vi "alignment_server_zmq.vi"() -> ()   [LabVIEW 2012]
uses:
  <vilib>/Platform/TimedLoop/XDataNode/wakeup.ctl
  <vilib>/Platform/TimedLoop/XDataNode/XDNodeRunTimeDep.lvlib
  <vilib>/Platform/TimedLoop/XDataNode/nitl_modes.ctl
  <vilib>/Platform/TimedLoop/XDataNode/timing_clust.ctl
  <vilib>/platform/TimedLoop/XDataNode/XDataNode.xnode
  Analog_Input/Analog_Input.lvclass
  PicoMotor.lvclass
  picomotor_control_array.ctl
  NewFocus8742/Command VIs/picomotor_control.ctl
  <vilib>/addons/zeromq/socket_type.ctl
panel:
  in  "enable":bool[](array[boolean])=[TRUE, TRUE, TRUE, TRUE]
  out "stopped?":bool[](array[boolean])
  out "Actual Positions":i32[](array[numeric])
  in  "Set Positions":i32[](array[numeric])=[0, 0, 0, 0] step=10
  in  "samples per channel":i32=100
  out "RECV'd message":string
  in  "Picomotor controls":T1=[{"enable"=TRUE, "description"="x1", "Set Position "=0, "Actual Position"=0, "stopped?"=TRUE, "zero"=FALSE, "Motor Type"=3, "Steps/s"=1750, "Steps/s^2"=100000}, {"enable"=TRUE, "description"="x2", "Set Position "=0, "Actual Position"=0, "stopped?"=TRUE, "zero"=FALSE, "Motor Type"=3, "Steps/s"=1750, "Steps/s^2"=100000}, {"enable"=TRUE, "description"="x3", "Set Position "=0, "Actual Position"=0, "stopped?"=TRUE, "zero"=FALSE, "Motor Type"=3, "Steps/s"=1750, "Steps/s^2"=100000}, {"enable"=TRUE, "description"="x4", "Set Position "=0, "Actual Position"=0, "stopped?"=TRUE, "zero"=FALSE, "Motor Type"=3, "Steps/s"=1750, "Steps/s^2"=100000}] {"Motor Type" items=["NoMotor", "Undefined", "Tiny", "Standard"]; "Set Position" step=100}
  in  "shutdown":bool caption="quit"
  in  "halt":bool caption="quit"
  out "voltage":dbl[](array[numeric])=[1.3462267936011734]
  out "coupling chart":dbl(graph)
  in  "descriptions":string[](array[string])
  out "DeviceKey Out":string="8742 10116"
  in  "sample rate (Hz)":dbl=1000.0
  in  "physical channels":tag="PXI1Slot7/ai0"
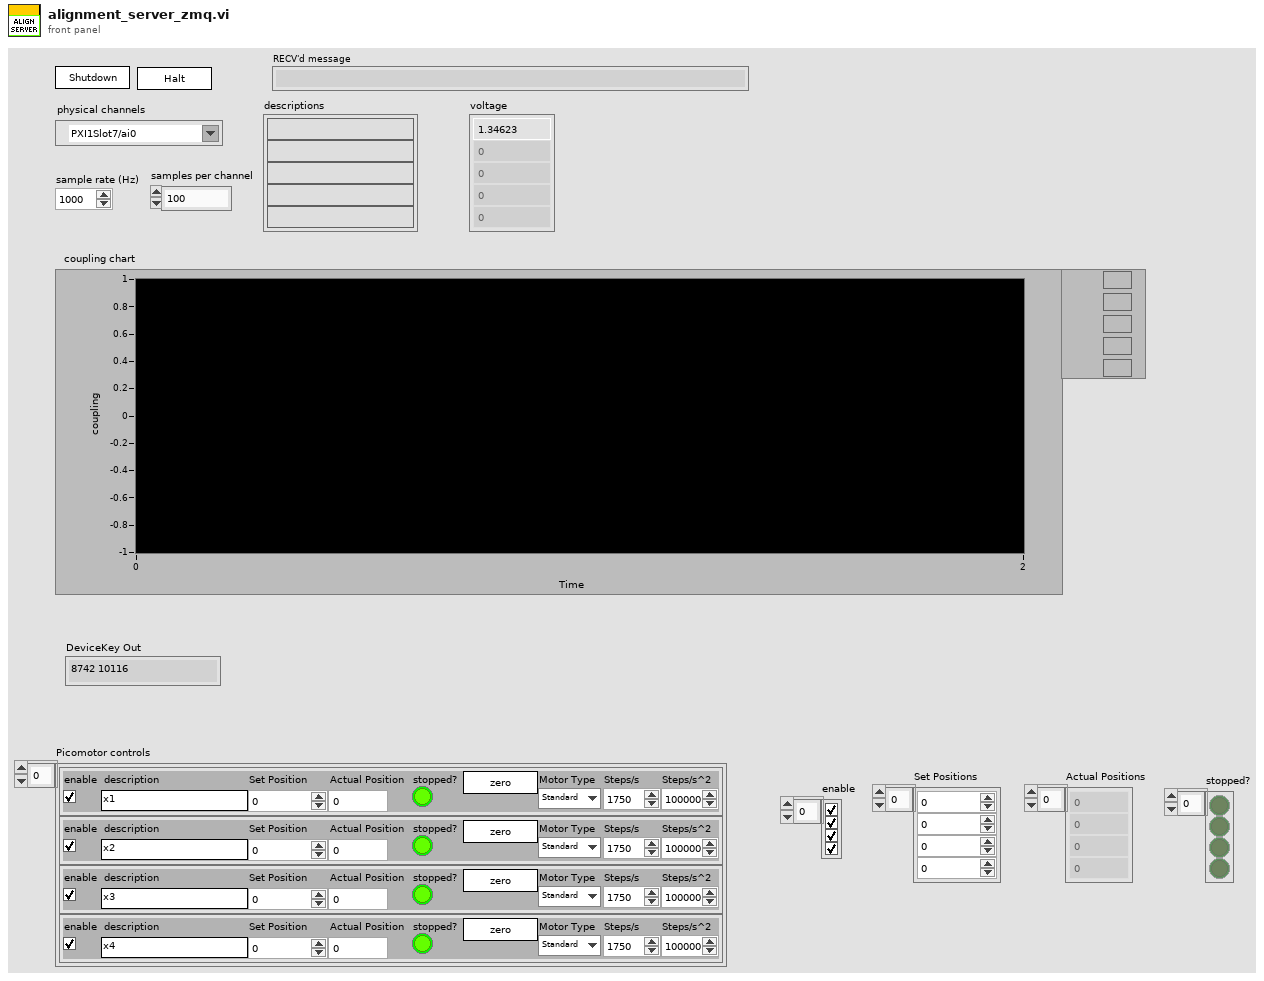
[diagram p1: front panel]
types:
  T1 = typedef "PicoMotor.lvclass/picomotor_control_array.ctl" = T2[]
  T2 = typedef "PicoMotor.lvclass/picomotor_control.ctl" = cluster{"enable":bool, "description":string, "Set Position ":i32, "Actual Position":i32, "stopped?":bool, "zero":bool, "Motor Type":i32, "Steps/s":i32, "Steps/s^2":i32}
  T3 = typedef "zeromq.lvlib/socket_type.ctl" = enum8{"ZMQ_PAIR", "ZMQ_PUB", "ZMQ_SUB", "ZMQ_REQ", "ZMQ_REP", "ZMQ_DEALER", "ZMQ_ROUTER", "ZMQ_PULL", "ZMQ_PUSH", "ZMQ_XPUB", "ZMQ_XSUB"}
  T4 = typedef "XDNodeRunTimeDep.lvlib/timing_clust.ctl" = cluster{"Expected End [f-1]":u64, "Actual End [f-1]":u64, "Finished Late? [f-1]":bool, "Expected End [i-1]":u64, "Actual End [i-1]":u64, "Finished Late? [i-1]":bool, "Expected Start [i]":u64, "Actual Start [i]":u64, "Expected Start [f]":u64, "Actual Start [f]":u64, "Source Name":string, "Structure Name":string, "Period":i64, "Deadline":i64, "Offset":i64, "Start":i64, "Priority":i32, "Timeout":i32, "Mode":T5, "Wakeup Reason":T6, "Error":errorcluster, "Source Type":string, "Secondary Source Type":string, "Global End Time":u64, "Global Start Time":u64, "Frame Duration":u64, "Iteration Duration":u64, "Assigned CPU":i32, "I/O Scan Engine Mode":u32}
  T5 = typedef "XDNodeRunTimeDep.lvlib/nitl_modes.ctl" = enum32{"No Change", "Process missed periods, maintain original phase", "Discard missed periods, maintain original phase", "Process missed periods, ignore original phase", "Discard missed periods, ignore original phase"}
  T6 = typedef "XDNodeRunTimeDep.lvlib/wakeup.ctl" = enum32{"Normal", "Aborted", "Asynchronous wakeup", "Timing source error", "Timed loop error", "Timeout"}
  T7 = typedef "pointer.ctl" = u64
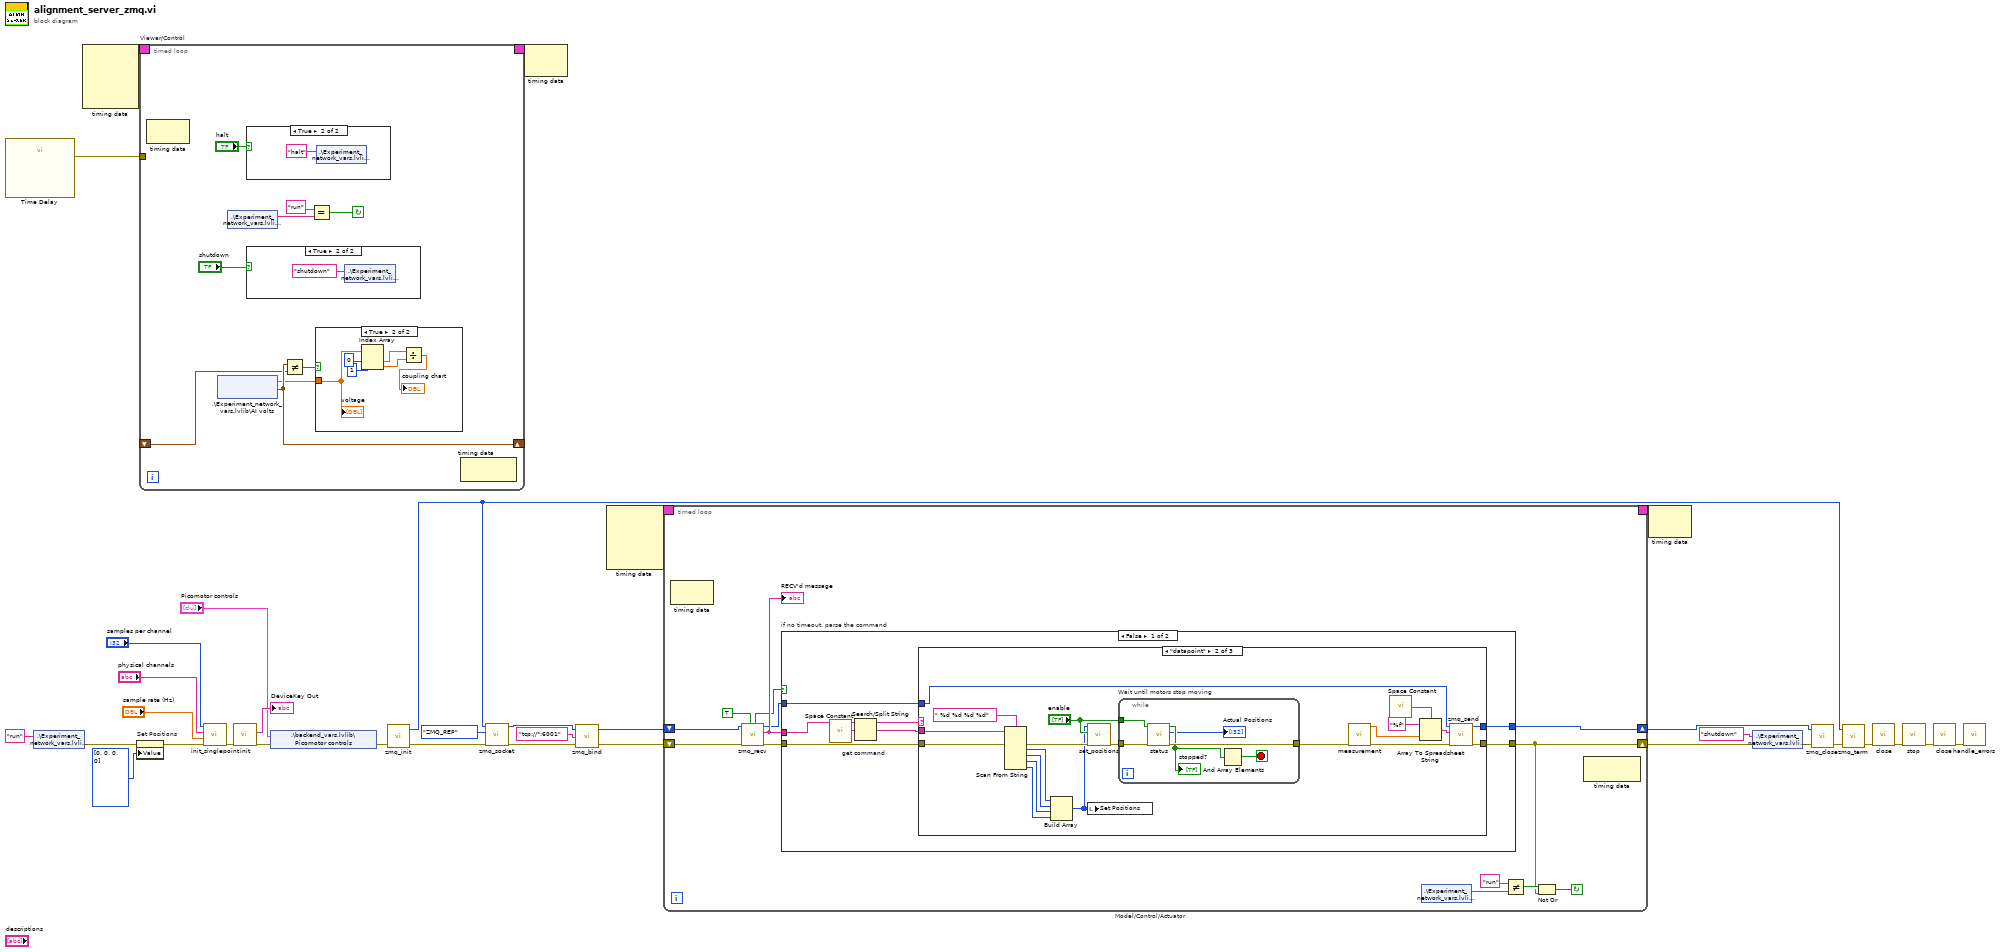
[diagram p0: block diagram]
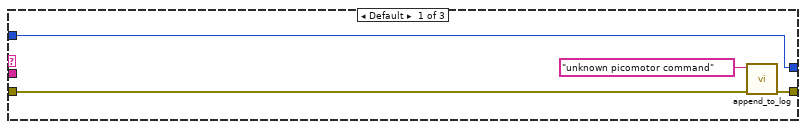
[diagram p2: hidden frame]
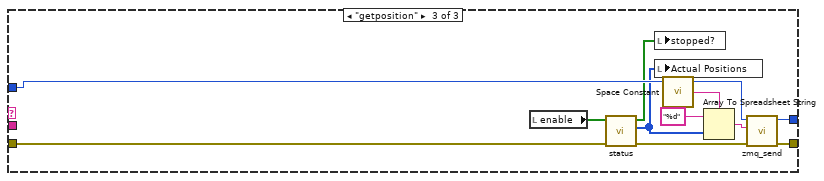
[diagram p3: hidden frame]
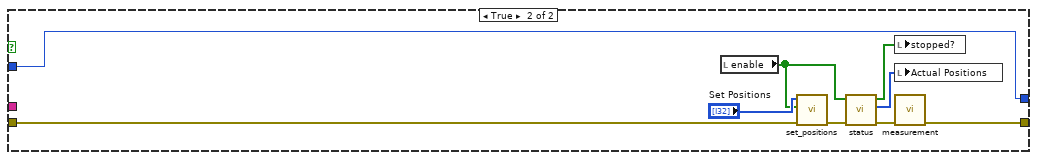
[diagram p4: hidden frame]
diagram:
  n1 = call "Time Delay"() -> ("error out"=w8:errorcluster)  [unwired: 11 in]
  n2 = shared-variable ".\\Experiment_network_vars.lvlib\\state"("run" ("state")) -> (error out=w3:errorcluster)  [unwired: 1 in]
  n3 = node-c288() -> (w34:T4)  [unwired: 4 in]
  n4 = property on="Set Positions" class="Arr (strict)"(error in=w3, "Value"=i32[] [0, 0, 0, 0] ("Set Positions")) -> (error out=w2:errorcluster)  [unwired: 1 in, 1 out]
  n5 = timed-loop "Viewer/Control" {
    timing: w34 -> [_]
    timing-out: [_] -> w33
    tunnel: w8 -> [_]
    shift-right: [w38] -> _
    shift-left: _ -> [w37]
    stop <- w39 continue-if-true
    n6 = node-c288() -> ()  [unwired: 1 in, 1 out]
    n7 = shared-variable ".\\Experiment_network_vars.lvlib\\AI volts"() -> (w35:dbl[], w38:timestamp)  [unwired: 1 in, 1 out]
    n8 = shared-variable ".\\Experiment_network_vars.lvlib\\state"() -> (w41:string)  [unwired: 1 in, 1 out]
    n9 = case shown="True" "halt" {
      frame False {
      }
      frame True {
        n10 = shared-variable ".\\Experiment_network_vars.lvlib\\state"("halt" ("state")) -> ()  [unwired: 1 in, 1 out]
      }
    }
    n11 = case shown="True" "shutdown" {
      frame False {
      }
      frame True {
        n12 = shared-variable ".\\Experiment_network_vars.lvlib\\state"("shutdown" ("state")) -> ()  [unwired: 1 in, 1 out]
      }
    }
    n13 = Not Equal?(x=w38, y=w37) -> (x != y?=w36:bool)
    n14 = Equal?(x="run", y=w41) -> (x = y?=w39:bool)
    n15 = case shown="True" w36 {
      tunnel: w35 -> [_ w48]
      frame False {
      }
      frame True {
        n16 = Index Array(array=w48, index #1=0 ("index"), index #2=1 ("index")) -> (element #1=w46:dbl, element #2=w45:dbl)
        n17 = Divide(x=w46, y=w45) -> (x/y=→"coupling chart":dbl)
        "voltage" <- w48
      }
    }
    n18 = node-c288() -> ()  [unwired: 1 in, 1 out]
  }
  n19 = call "init_singlepoint.vi"("error in"=w2, "sample rate (Hz)"="sample rate (Hz)", "physical channels"="physical channels", "samples per channel"="samples per channel") -> ("error out"=w5:errorcluster)  [unwired: 7 in]
  n20 = call "init.vi"("error in (no error)"=w5) -> ("error out"=w18:errorcluster, "DeviceKey"=→"DeviceKey Out":string)  [unwired: 9 in]
  n21 = shared-variable ".\\backend_vars.lvlib\\Picomotor controls"("Picomotor controls", error in=w18) -> (error out=w16:errorcluster)
  n22 = call <vilib>:"zmq_init.vi"("error in"=w16) -> ("error out"=w25:errorcluster, "context"=w23:T7)  [unwired: 3 in]
  n23 = call <vilib>:"zmq_socket.vi"("error in"=w25, "socket type"=socket_type."ZMQ_REP", "ctx in"=w23) -> ("error out"=w12:errorcluster, "socket"=w10:T7)  [unwired: 3 in]
  n24 = node-c288(w33) -> ()  [unwired: 1 out]
  n25 = call <vilib>:"zmq_bind.vi"("error in"=w12, "endpoint"="tcp://*:6001", "socket in"=w10) -> ("error out"=w11:errorcluster, "socket out"=w9:T7)  [unwired: 1 in]
  n26 = node-c288() -> (w32:T4)  [unwired: 4 in]
  n27 = timed-loop "Model/Control/Actuator" {
    timing: w32 -> [_]
    timing-out: [_] -> w31
    shift-right: [w62] -> w20
    shift-left: w9 -> [w61]
    shift-right: [w54] -> w14
    shift-left: w11 -> [w66]
    stop <- w57 continue-if-true
    n28 = node-c288() -> ()  [unwired: 1 in, 1 out]
    n29 = call <vilib>:"zmq_recv.vi"("no block? (F)"=TRUE, "error in"=w66, "socket in"=w61) -> ("error out"=w55:errorcluster, "data"=w64:string, "socket out"=w63:T7, "timeout?"=w56:bool)  [unwired: 2 in, 1 out]
    "RECV'd message" <- w64
    n30 = case "if no timeout, parse the command" shown="False" w56 {
      tunnel: [w71 w124] -> w54
      tunnel: w64 -> [w73 _]
      tunnel: w63 -> [w69 w123]
      tunnel: [w68 w123] -> w62
      tunnel: w55 -> [w67 w119]
      frame False {
        n31 = call <vilib>:"Space Constant.vi"() -> ("String"=w74:string)
        n32 = Search/Split String "get command"(string=w73, search string/char (-)=w74) -> (substring before match=w72:string, match + rest of string=w70:string)  [unwired: 1 in, 1 out]
        n33 = case shown="\"datapoint\"" w72 {
          tunnel: w67 -> [w77 w96 w115]
          tunnel: [w76 w88 w109] -> w71
          tunnel: w70 -> [_ w97 _]
          tunnel: w69 -> [w75 w90 w111]
          tunnel: [w75 w89 w108] -> w68
          frame Default {
            n34 = call "append_to_log.vi"("error in"=w77, "string"="unknown picomotor command") -> ("error out"=w76:errorcluster)  [unwired: 8 in, 1 out]
          }
          frame "datapoint" {
            n35 = Scan From String(format string=" %d %d %d %d", input string=w97, error in=w96) -> (error out=w81:errorcluster, output 1=w95:i32, output 2=w94:i32, output 3=w93:i32, output 4=w92:i32)  [unwired: 5 in, 2 out]
            n36 = Build Array(w95, w94, w93, w92) -> (w79:i32[])
            n37 = call "set_positions.vi"("error IO"=w81, "enables"="enable", "set positions"=w79) -> ("error out"=w82:errorcluster)  [unwired: 8 in]
            n38 = local write "Set Positions"(w79) -> ()
            n39 = while "Wait until motors stop moving" {
              tunnel: w82 -> [w104]
              tunnel: [w102] -> w91
              tunnel: "enable" -> [w101]
              stop <- w103 stop-if-true
              n40 = call "status.vi"("error IO"=w104, "enable"=w101) -> ("error out"=w102:errorcluster, "Actual Positions"=→"Actual Positions":i32[], "stopped?"=w100:bool[])  [unwired: 7 in]
              "stopped?" <- w100
              n41 = And Array Elements(Boolean array=w100) -> (logical AND=w103:bool)
            }
            n42 = call "measurement.vi"("error in"=w91) -> ("AI Volts"=w87:dbl[], "error out"=w83:errorcluster)  [unwired: 13 in]
            n43 = call <vilib>:"Space Constant.vi"() -> ("String"=w85:string)
            n44 = Array To Spreadsheet String(delimiter (Tab)=w85, array=w87, 3:"%f" ("format string")) -> (spreadsheet string=w84:string)
            n45 = call <vilib>:"zmq_send.vi"("error in"=w83, "data"=w84, "socket in"=w90) -> ("error out"=w88:errorcluster, "socket out"=w89:T7)  [unwired: 4 in]
          }
          frame "getposition" {
            n46 = local read "enable"() -> (w107:bool[])
            n47 = call "status.vi"("error IO"=w115, "enable"=w107) -> ("error out"=w110:errorcluster, "Actual Positions"=w105:i32[], "stopped?"=w106:bool[])  [unwired: 7 in]
            n48 = local write "stopped?"(w106) -> ()
            n49 = local write "Actual Positions"(w105) -> ()
            n50 = call <vilib>:"Space Constant.vi"() -> ("String"=w114:string)
            n51 = Array To Spreadsheet String(delimiter (Tab)=w114, array=w105, 3:"%d" ("format string")) -> (spreadsheet string=w112:string)
            n52 = call <vilib>:"zmq_send.vi"("error in"=w110, "data"=w112, "socket in"=w111) -> ("error out"=w109:errorcluster, "socket out"=w108:T7)  [unwired: 4 in]
          }
        }
      }
      frame True {
        n53 = local read "enable"() -> (w116:bool[])
        n54 = call "set_positions.vi"("error IO"=w119, "enables"=w116, "set positions"="Set Positions") -> ("error out"=w118:errorcluster)  [unwired: 8 in]
        n55 = call "status.vi"("error IO"=w118, "enable"=w116) -> ("error out"=w122:errorcluster, "Actual Positions"=w120:i32[], "stopped?"=w121:bool[])  [unwired: 7 in]
        n56 = local write "stopped?"(w121) -> ()
        n57 = local write "Actual Positions"(w120) -> ()
        n58 = call "measurement.vi"("error in"=w122) -> ("error out"=w124:errorcluster)  [unwired: 13 in, 1 out]
      }
    }
    n59 = shared-variable ".\\Experiment_network_vars.lvlib\\state"() -> (w60:string)  [unwired: 1 in, 1 out]
    n60 = Not Equal?(x="run", y=w60) -> (x != y?=w58:bool)
    n61 = Not Or(1:w54, 2:w58) -> (0:w57:bool)
    n62 = node-c288() -> ()  [unwired: 1 in, 1 out]
  }
  n63 = node-c288(w31) -> ()  [unwired: 1 out]
  n64 = shared-variable ".\\Experiment_network_vars.lvlib\\state"("shutdown" ("state"), error in=w14) -> (error out=w21:errorcluster)
  n65 = call <vilib>:"zmq_close.vi"("error in"=w21, "socket in"=w20) -> ("error out"=w24:errorcluster)  [unwired: 3 in]
  n66 = call <vilib>:"zmq_term.vi"("error in"=w24, "context"=w23) -> ("error out"=w19:errorcluster)  [unwired: 3 in]
  n67 = call "close.vi"("error IO"=w19) -> ("error"=w26:errorcluster)  [unwired: 10 in]
  n68 = call "stop.vi"("error in (no error)"=w26) -> ("error out"=w29:errorcluster)  [unwired: 10 in]
  n69 = call "close.vi"("error in (no error)"=w29) -> ("error out"=w28:errorcluster)  [unwired: 10 in]
  n70 = call "handle_errors.vi"("error in (no error)"=w28) -> ()  [unwired: 9 in, 2 out]
